vi "ActorPlugin-002-Inventory.vi"(0 "FTW Actor Instance Configuration":string="{\n  \"Identity\": \"ActorName\",\n  \"InboxAddress\": \"tcp://127.0.0.1:*\",\n  \"PublisherAddress\": \"tcp://127.0.0.1:*\",\n  \"DebugEnableInboxLogging\": false,\n  \"DebugEnableJobLogging\": false,\n  \"DebugShowPanel\": false\n}", 11 "Error":errorcluster) -> (15 "Error":errorcluster)   [LabVIEW 2013, in "ERP-Inventory.lvclass"]
uses:
  Actors/ERP-Inventory Plugin/ERP-Inventory.lvclass
  Inventory System/controls/Create Label Button.ctl
  Actors/ERP-Inventory Plugin/Inventory-Controls/Iventory-FinishedGoods.ctl
  Actors/ERP-Inventory Plugin/Inventory-Controls/Iventory-RawGoods.ctl
  Actors/ERP-Inventory Plugin/Inventory-Controls/Iventory-AdminOnly.ctl
  Actors/ERP-Inventory Plugin/ERP-Inventory.lvclass/ERP-Inventory.ctl
  <vilib>/Utility/error.llb/DialogType.ctl
  <vilib>/Utility/miscctls.llb/LVRowAndColumnUnsignedTypeDef.ctl
  ftw-dataflow/Actor/src/Instance/FTW-ActorInstance.lvclass
  ftw-dataflow/Actor/src/Message/Request/FTW-Message-IncomingRequest.lvclass
  ERP-ConfigPageNewFeather/PCert-ConfigPageNF.lvclass
panel:
  in  "Create Bag Label":T1
  in  "Admin":T2
  in  "Raw Goods":T3
  in  "Finished Goods":T4
  in  "Tab Control - Finished Goods":T5(tab)
  in  "Quanity to Add/Subtract":i32
  in  "Part Number to Search For":string
  in  "Refresh Finished Good List":bool
  in  "Clear Search":bool
  in  "Search Button":bool
  in  "Inventory Listbox":i32(listbox)
  in  "Add Finshed Goods":bool
  in  "Part Numbers":u16(ring) items=["", "------------Wafers---------------", "PC-1012MX", "PC-1015M", "PP-2015-7003SCM", "PP-2015-9903SC/I-M", "PP-2015-15003SCM", "PP-2023-7003SCM", "PP-2023-15003SCM", "PP-2023-30003SCM", "PL-5015-05AH", "PL-5015-1AH", "PL-5023-1AHG", "PF-4015-30003SCM", "PF-4022-30003SCM", "PF-4023-30003SCM", "PF-4043-30003SCM", "PF-4043-30015SCM", "-------Miscelaneous Parts-------", "TPR-CRP", "TPR-VRP", "TPR-LPF05", "TPR-LPF10", "TPR-VLPF-3SH", "PL-5001-1AH", "PP-2001-7003SCM", "PP-2001-9903SC/I-M", "PS-3001-1AHM", "PF-4001-30003SCM", "PP-2010-7003SCM", "PL-5010-1AH", "PS-3010-3AHM", "PF-4010-30015SCM", "PP-2049-30003SCM", "PP-2049-7003SCM", "PL-5049-1AH", "PP-2049-7003SCM", "PL-5044-1AH", "PL-5121-1AH", "PP-2055-7003SCM", "PL-5055-1AH", "PP-2129-7003SCM", "PL-5338-1AH", "PF-4014-30003SCM", "PF-4014-30010SCM", "PF-4008-30015SCM", "PF-4064-30015SCM", "PF-4111-30003SCM", "PF-4054-30003SCM", "NS-PP-2150-15003SCM", "CCW-7015-001-257-FL", "CCW-7015-01-150-FL", "CCW-7043-001-257-FL", "CCW-7043-01-150-FL", "Vacuum Chuck", "HHCR-12-1"]
  in  "Subtract Finished Goods":bool
  in  "Part Number to Search For Raw Goods":string caption="Part Number to Search For"
  in  "Subtract_Raw Goods":bool
  in  "Quanity to Add/Subtract_Raw Goods":i32 caption="Quanity to Add/Subtract"
  in  "Part Numbers_Raw Goods":u16(ring) caption="Part Numbers" items=["", "X042-MJC", "X042-IMFS", "X043-ITS", "X043J-ITS", "X022-ITS", "X023-ITS", "X016-MJC", "X094-ITS", "X094-TI", "X015-IMFT", "X015-MJC", "X015-ITS"]
  in  "Add Button_Raw Goods":bool
  in  "Raw Goods Listbox":i32(listbox)
  in  "Search Button_Raw Goods":bool
  in  "Clear Search_Raw Goods":bool
  in  "Refresh Raw Good List":bool
  in  "Tab Control - Delete Part Numbers":enum32{"Finsihed Goods", "Raw Goods"}(tab)
  in  "Delete Finished Good Part Number":bool
  in  "Finish Good Part# to Delete":u16(ring) caption="Part Numbers" items=["", "------------Wafers---------------", "PC-1012MX", "PC-1015M", "PP-2015-7003SCM", "PP-2015-9903SC/I-M", "PP-2015-15003SCM", "PP-2023-7003SCM", "PP-2023-15003SCM", "PP-2023-30003SCM", "PL-5015-05AH", "PL-5015-1AH", "PL-5023-1AHG", "PF-4015-30003SCM", "PF-4022-30003SCM", "PF-4023-30003SCM", "PF-4043-30003SCM", "PF-4043-30015SCM", "-------Miscelaneous Parts-------", "TPR-CRP", "TPR-VRP", "TPR-LPF05", "TPR-LPF10", "TPR-VLPF-3SH", "PL-5001-1AH", "PP-2001-7003SCM", "PP-2001-9903SC/I-M", "PS-3001-1AHM", "PF-4001-30003SCM", "PP-2010-7003SCM", "PL-5010-1AH", "PS-3010-3AHM", "PF-4010-30015SCM", "PP-2049-30003SCM", "PP-2049-7003SCM", "PL-5049-1AH", "PP-2049-7003SCM", "PL-5044-1AH", "PL-5121-1AH", "PP-2055-7003SCM", "PL-5055-1AH", "PP-2129-7003SCM", "PL-5338-1AH", "PF-4014-30003SCM", "PF-4014-30010SCM", "PF-4008-30015SCM", "PF-4064-30015SCM", "PF-4111-30003SCM", "PF-4054-30003SCM", "NS-PP-2150-15003SCM", "CCW-7015-001-257-FL", "CCW-7015-01-150-FL", "CCW-7043-001-257-FL", "CCW-7043-01-150-FL", "Vacuum Chuck", "HHCR-12-1"]
  in  "Raw Goods Part # to Delete":u16(ring) caption="Part Numbers" items=["", "X042-MJC", "X042-IMFS", "X043-ITS", "X043J-ITS", "X022-ITS", "X023-ITS", "X016-MJC", "X094-ITS", "X094-TI", "X015-IMFT", "X015-MJC", "X015-ITS"]
  in  "Delete Raw Good Part Number":bool
  in  "Maximum Number Allowed\nIn Inventory":i32
  in  "Minimum Number Allowed \nIn Inventory":i32
  in  "New Raw Good Part Number":bool
  in  "New Wafer Assembled Part?":bool
  in  "New Inventory Assembled Part Number to Add":string
  in  "Quanity to Add To Inventory New Part":i32
  out "String":string
  # "Inventory Controls"
  # "Inputs"
  # "Outputs"
  # "I am ready to run"
  # "Welcome to the ITS Inventory System\nPlease use the Inventory Controls below to \naccess the system."
  # "Finished Goods"
  # "Search Finished Goods DB"
  # "Add Part Number to Finished Goods"
  # "1."
  # "2."
  # "Raw Goods"
  # "Search Raw Goods DB"
  # "Add Part Number to Raw Goods"
  # "1."
  # "2."
  # "Admin Tools"
  # "Admin Add Parts to Database"
  # "Admin Delete Parts# From Database"
  # "Choose the Part Number that you would like to delete from the drop down menu. Then press delete."
  # "Choose the Part Number that you would like to delete from the drop down menu. Then press delete."
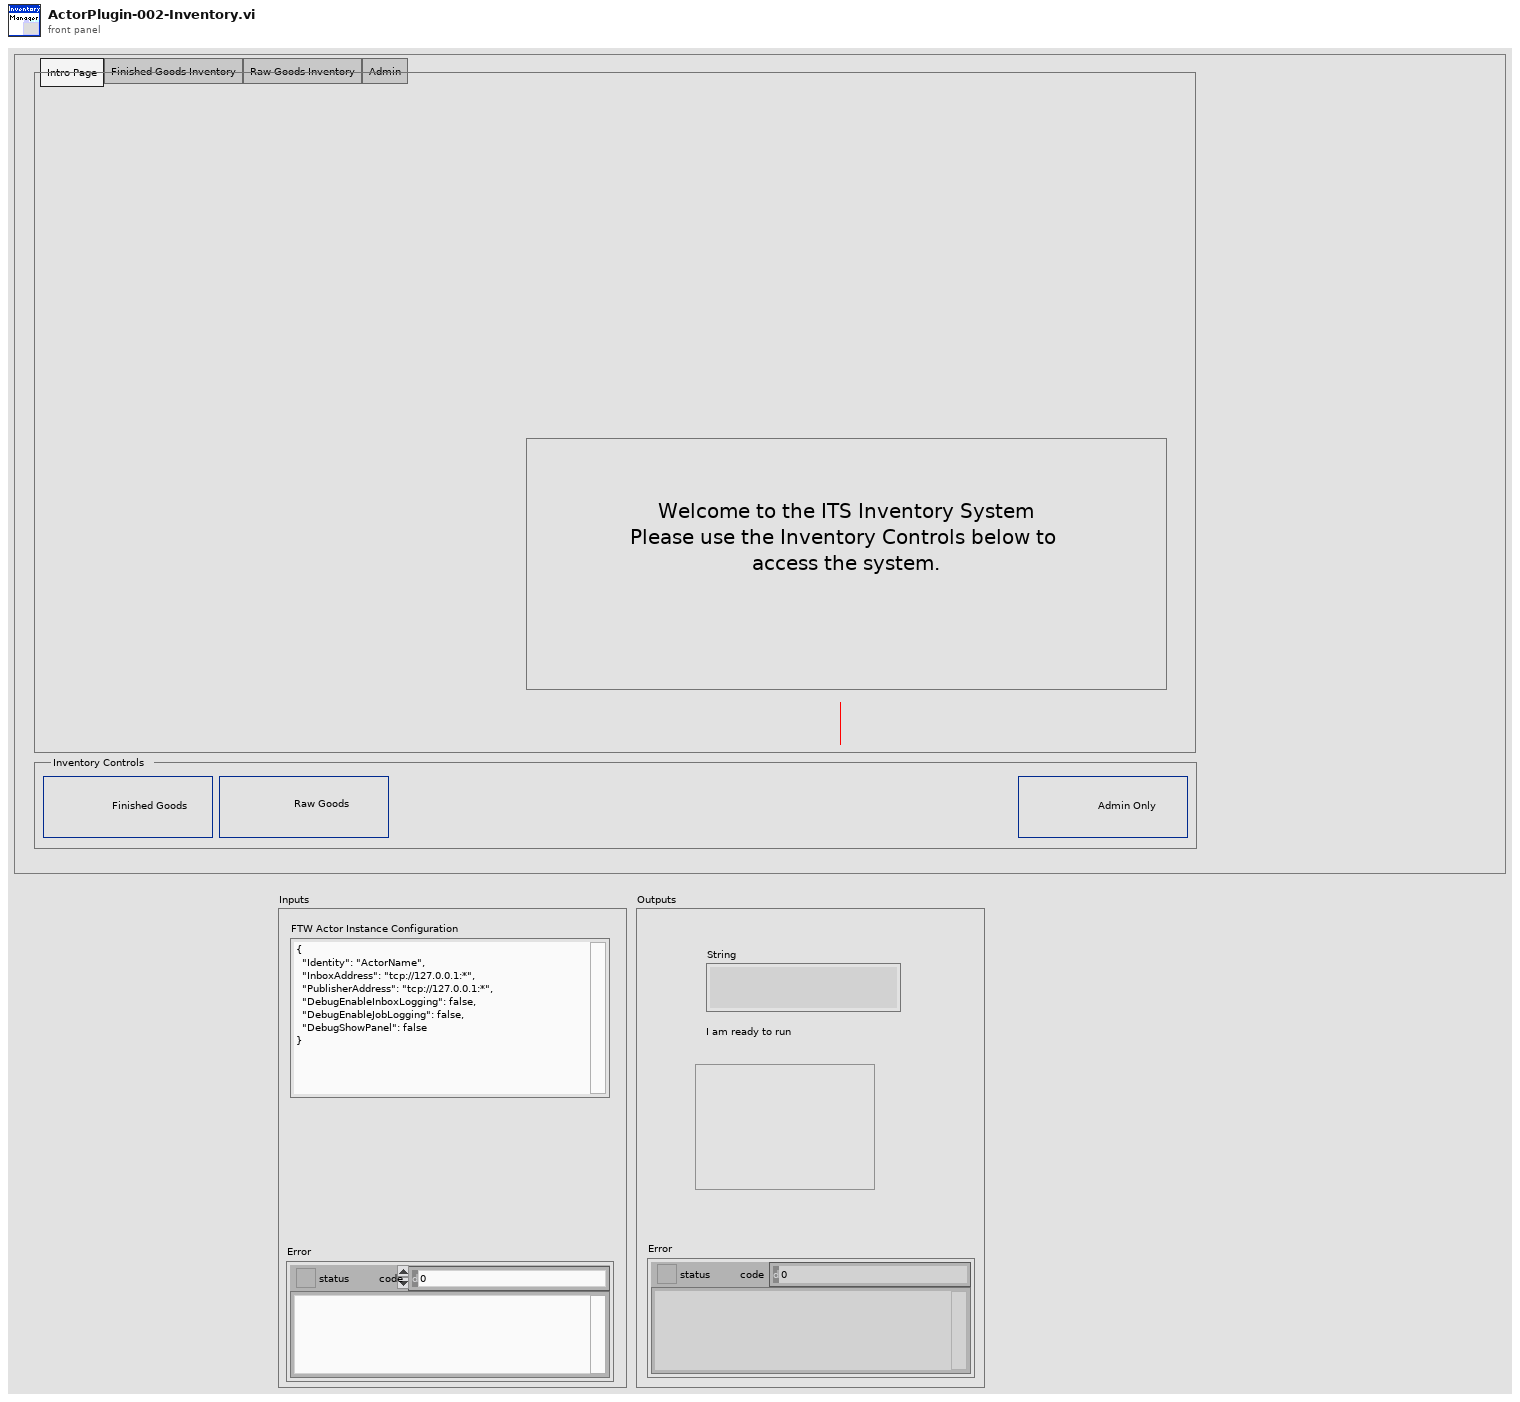
[diagram p1: front panel]
types:
  T1 = typedef "Create Label Button.ctl" = bool
  T2 = typedef "Iventory-AdminOnly.ctl" = bool
  T3 = typedef "Iventory-RawGoods.ctl" = bool
  T4 = typedef "Iventory-FinishedGoods.ctl" = bool
  T5 = enum32{"Intro Page", "Finished Goods Inventory", "Raw Goods Inventory", "Admin"}
  T6 = enum32{"Intro Page", "Finished Goods Inventory", "Raw Goods Inventory", "Inventory Waiting to be Stocked", "Fulfill Inventory Work Order", "Admin"}
  T7 = typedef "LVRowAndColumnUnsignedTypeDef.ctl" = cluster{"Row":u32, "Column":u32}
  T8 = cluster{"New Inventory Assembled Part Number to Add":string, "On the Shelf":string, "Minimum":string, "Maximum":string}
  T9 = typedef "DialogType.ctl" = u16
  T10 = cluster{"Incoming Requests":refnum<event-registration>, "Additional Registration Types":refnum<event-registration>}
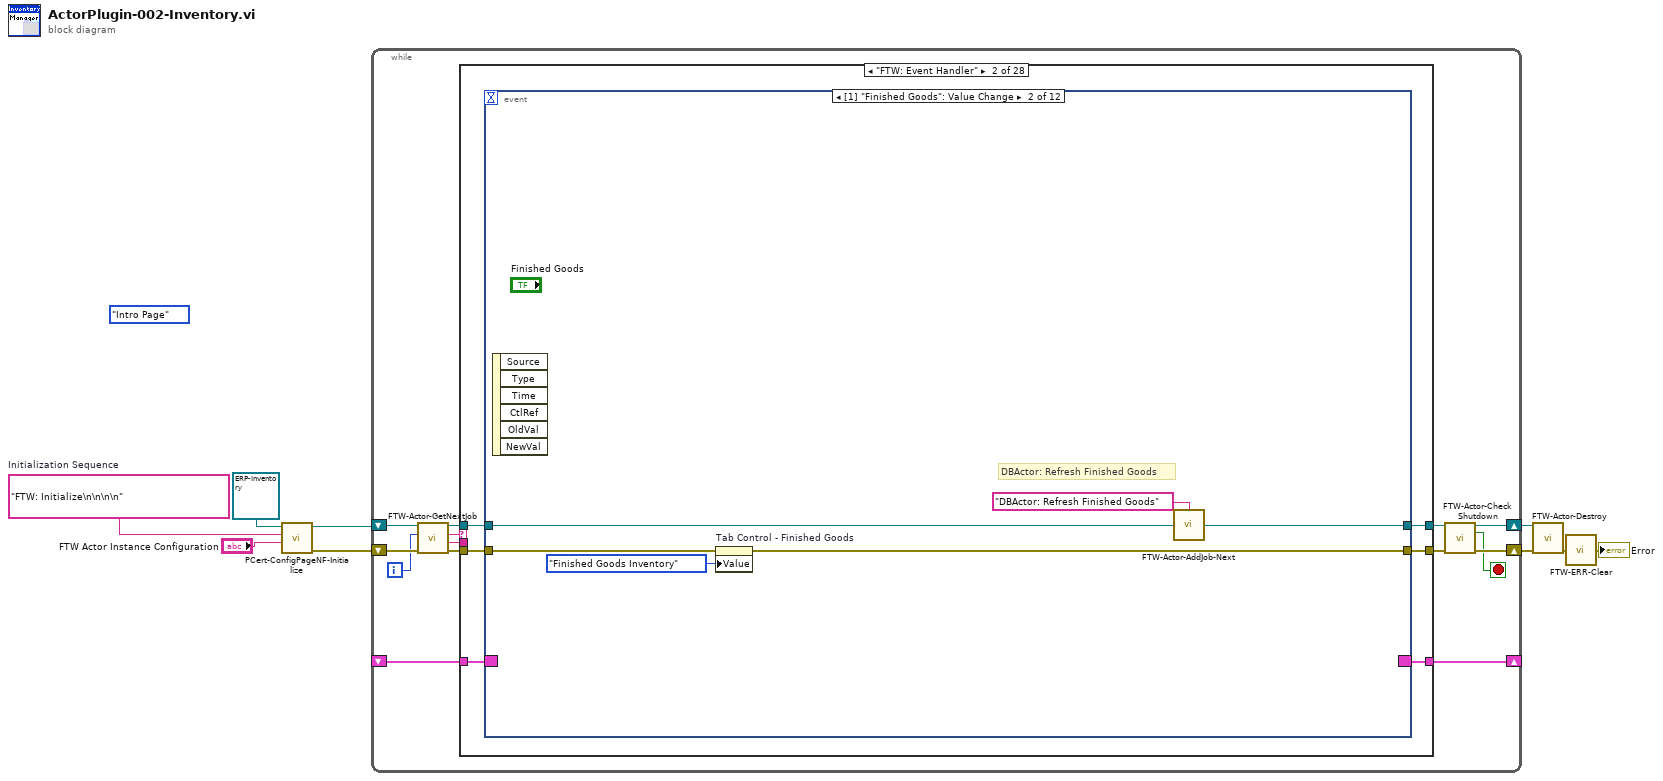
[diagram p0: block diagram]
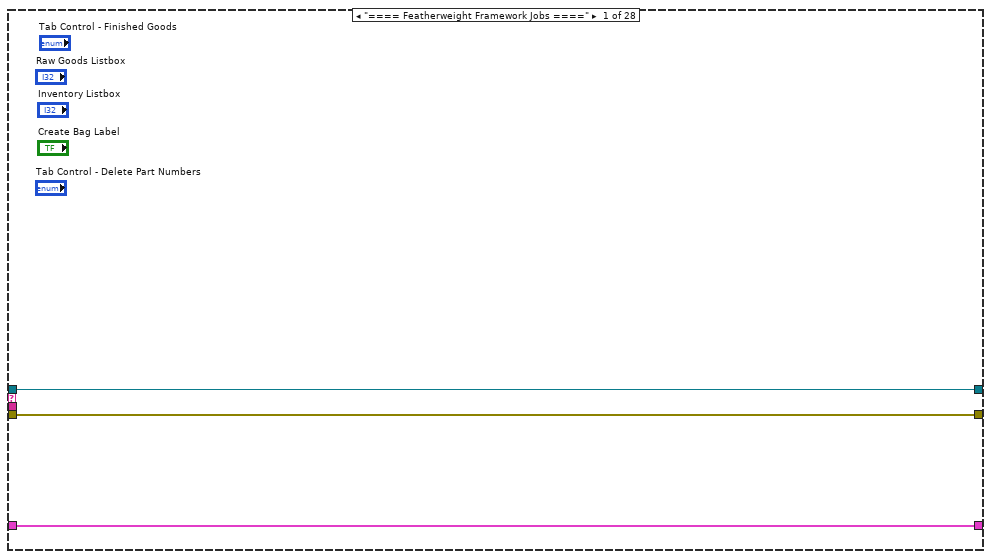
[diagram p2: hidden frame]
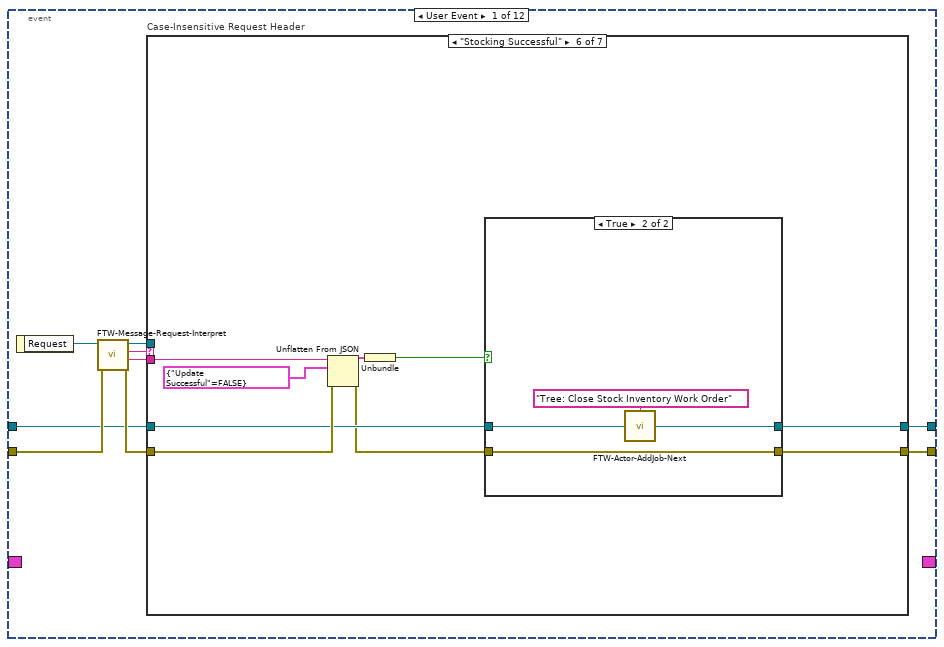
[diagram p3: hidden frame]
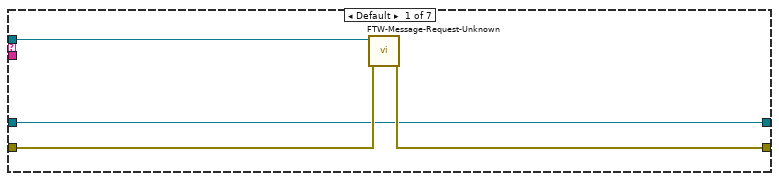
[diagram p4: hidden frame]
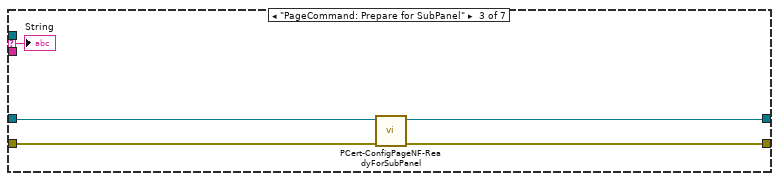
[diagram p6: hidden frame]
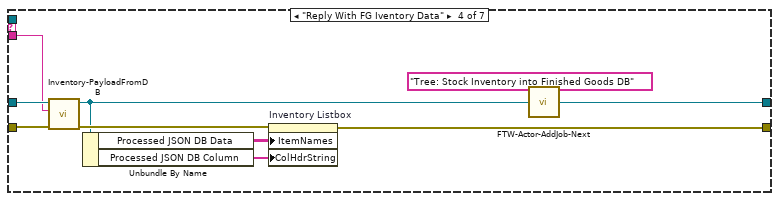
[diagram p7: hidden frame]
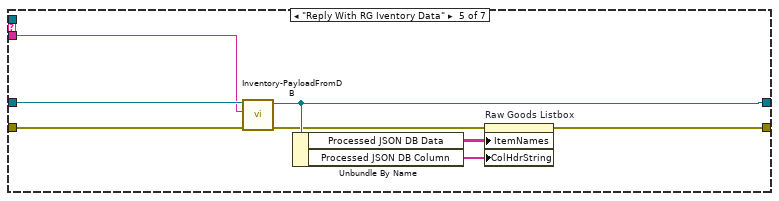
[diagram p8: hidden frame]
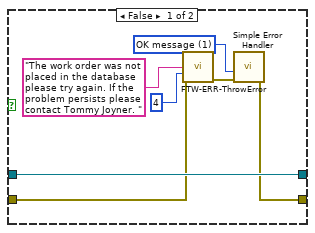
[diagram p9: hidden frame]
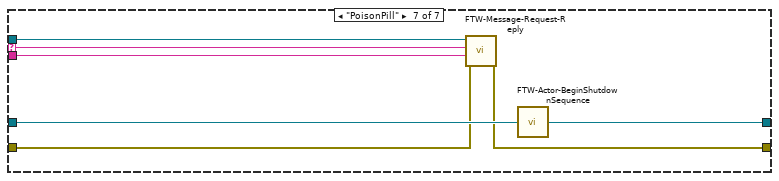
[diagram p10: hidden frame]
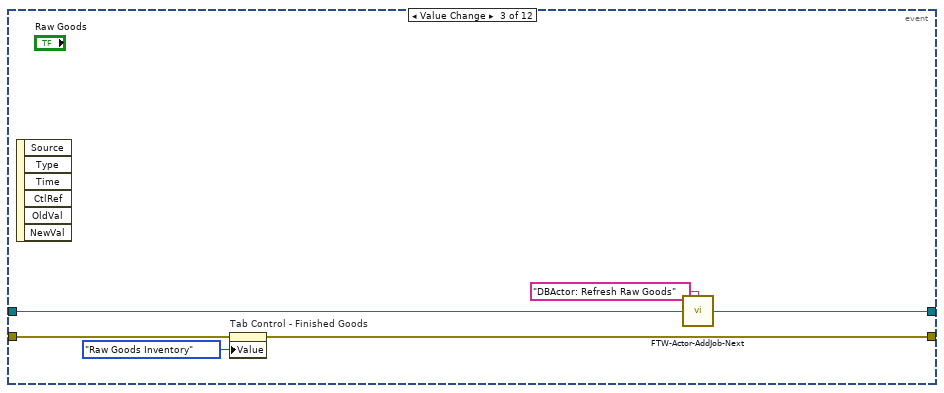
[diagram p11: hidden frame]
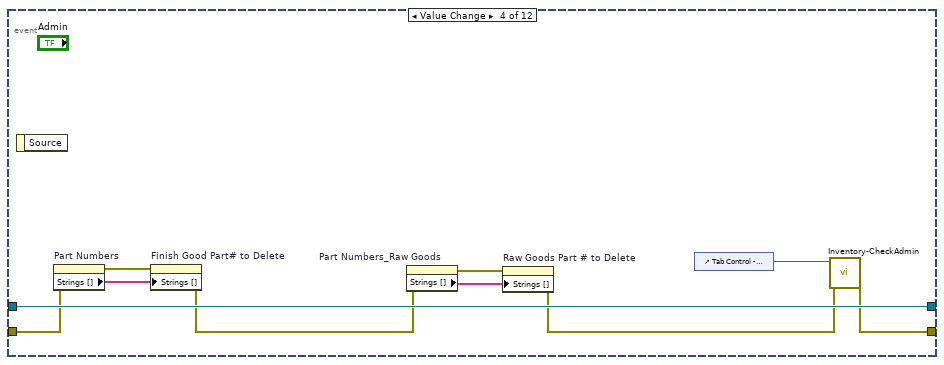
[diagram p12: hidden frame]
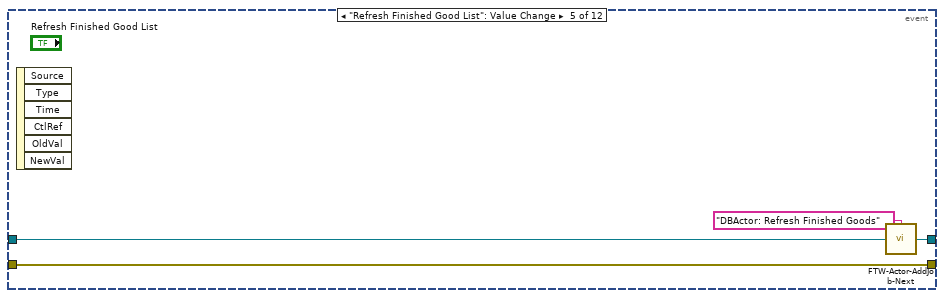
[diagram p13: hidden frame]
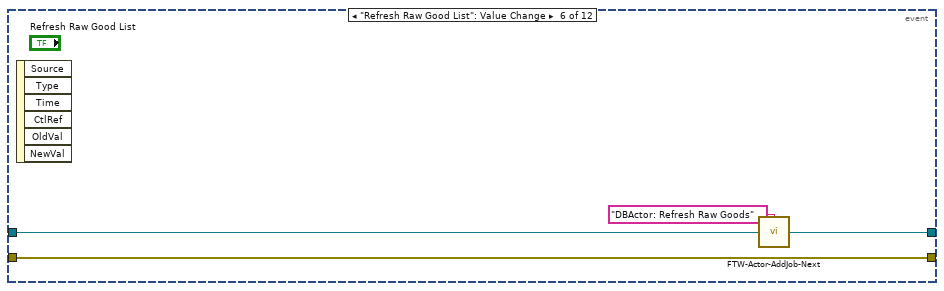
[diagram p14: hidden frame]
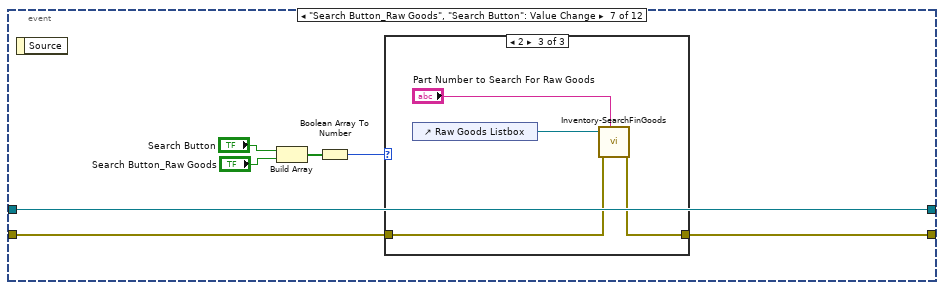
[diagram p15: hidden frame]
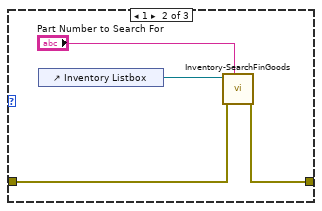
[diagram p17: hidden frame]
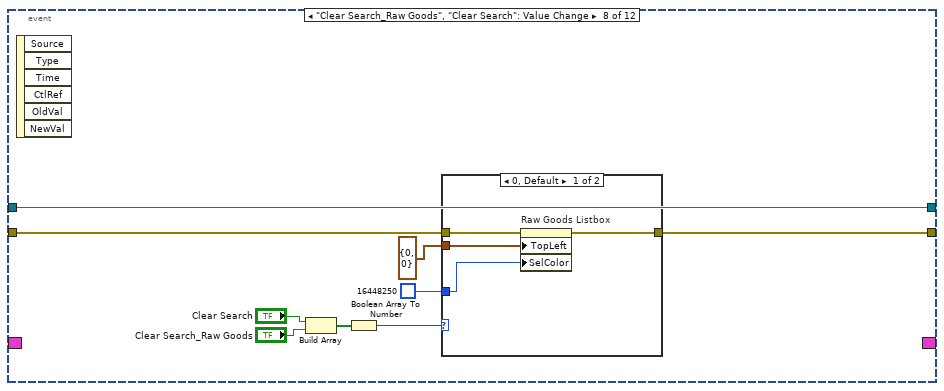
[diagram p18: hidden frame]
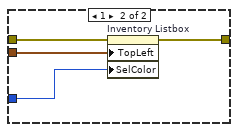
[diagram p19: hidden frame]
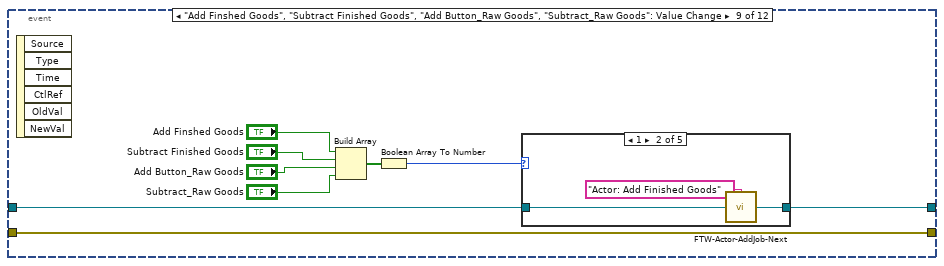
[diagram p20: hidden frame]
diagram:
  (unwired) T6."Intro Page" ("Tab Control - Finished Goods")
  w7 = "FTW: Initialize\n\n\n\n"  # Initialization Sequence
  n1 = call-dynamic "PCert-ConfigPageNF-Initialize.vi"("FTW Actor Instance Configuration"="FTW Actor Instance Configuration", "Initialization Job Sequence"=w7, "ERP-ConfigPageNF.lvclass"=refnum<class "ERP-Inventory.lvclass"> refnum ("ERP-Inventory.lvclass")) -> ("error out"=w5:errorcluster, "ERP-ConfigPageNF out"=w6:refnum<class "ERP-Inventory.lvclass">)  [unwired: 7 in]
  n2 = while {
    shift-right: [w13] -> w8
    shift-left: w5 -> [w20]
    shift-right: [w10] -> _
    shift-left: _ -> [w23]
    shift-right: [w15] -> w9
    shift-left: w6 -> [w22]
    i -> [w11]
    stop <- w12 stop-if-true
    n3 = call "FTW-Actor-GetNextJob.vi"("error in"=w20, "Jobs Performed"=w11, "FTW Actor Instance"=w22) -> ("error out"=w19:errorcluster, "Job Data"=w17:string, "Job Name"=w18:string, "FTW Actor Instance out"=w21:refnum<class "ERP-Inventory.lvclass">)  [unwired: 5 in]
    n4 = case shown="\"FTW: Event Handler\"" w18 {
      selector: w18 -> [_ _ _ _ w245 _ _ _ _ _ _ _ _ _ _ _ _ _ _ _ _ _ _ _ _ _ _ _]
      tunnel: [w25 w32 w238 w240 w248 w256 w262 w267 w271 w277 w292 w305 w320 w353 w386 w437 w486 w536 w566 w608 w632 w645 w648 w651 w654 w657 w660 w663] -> w14
      tunnel: w19 -> [w25 w31 w233 w242 w249 w252 w262 w267 w271 w283 w299 w314 w330 w342 w388 w439 w489 w558 w567 w604 w624 w645 w648 w651 w654 w657 w660 w663]
      tunnel: w23 -> [w26 w27 _ w244 w250 w258 w263 w268 w270 w287 w303 w319 w335 w361 w411 w461 w511 w565 w595 w619 w643 w646 w649 w652 w655 w658 w661 w664]
      tunnel: [w26 w30 w235 w244 w250 w258 w263 w268 w270 w287 w303 w319 w335 w361 w411 w461 w511 w565 w595 w619 w643 w646 w649 w652 w655 w658 w661 w664] -> w10
      tunnel: w17 -> [_ _ _ _ _ _ _ _ _ _ _ _ _ _ _ _ _ _ _ _ _ _ _ _ _ _ _ _]
      tunnel: [w24 w29 w239 w241 w246 w253 w260 w265 w269 w272 w288 w304 w321 w354 w387 w436 w487 w564 w568 w609 w633 w644 w647 w650 w653 w656 w659 w662] -> w16
      tunnel: w21 -> [w24 w28 w234 w243 w247 w254 w261 w266 w269 w279 w293 w309 w326 w360 w389 w438 w488 w559 w569 w610 w634 w644 w647 w650 w653 w656 w659 w662]
      frame "==== Featherweight Framework Jobs ====" {
      }
      frame "FTW: Event Handler" {
        n5 = event shown="[1] \"Finished Goods\": Value Change" {
          selector: w27 -> [_ _ _ _ _ _ _ _ _ _ _ _]
          dyn-events: [_ _ _ _ _ _ _ _ _ _ _ _] -> w30
          timeout: _ -> [_ _ _ _ _ _ _ _ _ _ _ _]
          tunnel: [w38 w102 w108 w118 w123 w127 w132 w150 w169 w183 w217 w227] -> w32
          tunnel: w31 -> [w39 w103 w109 w114 w123 w127 w133 w151 w169 w189 w217 w227]
          tunnel: [w37 w101 w106 w119 w121 w125 w134 w152 w161 w194 w213 w225] -> w29
          tunnel: w28 -> [w36 w99 w105 w119 w120 w124 w134 w152 w162 w200 w214 w226]
          event User Event {
            n6 = event-data() -> ("Request"=w40:refnum<class "FTW-Message-IncomingRequest.lvclass">)  [unwired: 1 in]
            n7 = call "FTW-Message-Request-Interpret.vi"("error in"=w39, "FTW Incoming Request"=w40) -> ("error out"=w41:errorcluster, "Request Body"=w34:string, "Request Header"=w35:string, "FTW Incoming Request out"=w33:refnum<class "FTW-Message-IncomingRequest.lvclass">)  [unwired: 6 in]
            n8 = case "Case-Insensitive Request Header" shown="\"Stocking Successful\"" w35 {
              selector: w35 -> [_ _ w48 _ _ _ w93]
              tunnel: [w44 w46 w50 w62 w66 w71 w91] -> w38
              tunnel: w41 -> [w45 w46 w52 w60 w69 w78 w92]
              tunnel: [w42 w47 w49 w54 w68 w73 w97] -> w37
              tunnel: w36 -> [w42 w47 w51 w61 w70 w74 w96]
              tunnel: w34 -> [_ _ _ w53 w63 w79 w94]
              tunnel: w33 -> [w43 _ _ _ _ _ w95]
              frame Default {
                n9 = call "FTW-Message-Request-Unknown.vi"("error in"=w45, "FTW Incoming Request"=w43) -> ("error out"=w44:errorcluster)  [unwired: 9 in]
              }
              frame "Cold Call Success" {
              }
              frame "PageCommand: Prepare for SubPanel" {
                n10 = call "PCert-ConfigPageNF-ReadyForSubPanel.vi"("error in (no error)"=w52, "ERP-ConfigPageNF in"=w51) -> ("error out"=w50:errorcluster, "ERP-ConfigPageNF out"=w49:refnum<class "ERP-Inventory.lvclass">)  [unwired: 8 in]
                "String" <- w48
              }
              frame "Reply With FG Iventory Data" {
                n11 = call "Inventory-PayloadFromDB.vi"("error in (no error)"=w60, "JSON string"=w53, "ERP-Inventory in"=w61) -> ("error out"=w59:errorcluster, "ERP-Inventory out"=w55:refnum<class "ERP-Inventory.lvclass">)  [unwired: 7 in]
                n12 = Unbundle By Name(w55) -> ("Processed JSON DB Data"=w58:string[][], "Processed JSON DB Column"=w57:string[])
                n13 = property on="Inventory Listbox" class="MCListbox (strict)"(error in=w59, "ItemNames"=w58, "ColHdrString"=w57) -> (error out=w62:errorcluster)  [unwired: 1 in, 1 out]
                n14 = call "FTW-Actor-AddJob-Next.vi"("Add Next in Job Queue"="Tree: Stock Inventory into Finished Goods DB", "FTW Actor Instance"=w55) -> ("FTW Actor Instance out"=w54:refnum<class "ERP-Inventory.lvclass">)  [unwired: 2 in]
              }
              frame "Reply With RG Iventory Data" {
                n15 = call "Inventory-PayloadFromDB.vi"("error in (no error)"=w69, "JSON string"=w63, "ERP-Inventory in"=w70) -> ("error out"=w67:errorcluster, "ERP-Inventory out"=w68:refnum<class "ERP-Inventory.lvclass">)  [unwired: 7 in]
                n16 = Unbundle By Name(w68) -> ("Processed JSON DB Data"=w65:string[][], "Processed JSON DB Column"=w64:string[])
                n17 = property on="Raw Goods Listbox" class="MCListbox (strict)"(error in=w67, "ItemNames"=w65, "ColHdrString"=w64) -> (error out=w66:errorcluster)  [unwired: 1 in, 1 out]
              }
              frame "Stocking Successful" {
                n18 = Unflatten From JSON(JSON string=w79, type and defaults=cluster{"Update Successful":bool} {"Update Successful"=FALSE}, error in (no error)=w78) -> (value=w76:cluster{"Update Successful":bool}, error out=w72:errorcluster)  [unwired: 4 in]
                n19 = Unbundle(w76) -> ("Update Successful"=w75:bool)
                n20 = case shown="True" w75 {
                  tunnel: w74 -> [w86 w89]
                  tunnel: [w86 w88] -> w73
                  tunnel: w72 -> [w82 w87]
                  tunnel: [w81 w87] -> w71
                  frame False {
                    w83 = T9 1 items=["no dialog", "OK message", "continue or stop message", "OK message + warnings", "continue/stop + warnings"] ("type of dialog (OK msg:1)")
                    n21 = call "FTW-ERR-ThrowError.vi"("Error Message"="The work order was not placed in the database please try again. If the problem persists please contact Tommy Joyner. ", "Error Code"=4, "error in"=w82) -> ("error out"=w84:errorcluster)  [unwired: 12 in]
                    n22 = call <vilib>:"Simple Error Handler.vi"("type of dialog (OK msg:1)"=w83, "error in (no error)"=w84) -> ("error out"=w81:errorcluster)  [unwired: 3 in, 4 out]
                  }
                  frame True {
                    n23 = call "FTW-Actor-AddJob-Next.vi"("Add Next in Job Queue"="Tree: Close Stock Inventory Work Order", "FTW Actor Instance"=w89) -> ("FTW Actor Instance out"=w88:refnum<class "ERP-Inventory.lvclass">)  [unwired: 2 in]
                  }
                }
              }
              frame "PoisonPill" {
                n24 = call "FTW-Message-Request-Reply.vi"("error in"=w92, "Response Body"=w94, "Response Header"=w93, "FTW Incoming Request"=w95) -> ("error out"=w91:errorcluster)  [unwired: 6 in, 1 out]
                n25 = call "FTW-Actor-BeginShutdownSequence.vi"("FTW Actor Instance"=w96) -> ("FTW Actor Instance out"=w97:refnum<class "ERP-Inventory.lvclass">)  [unwired: 3 in]
              }
            }
          }
          event Value Change {
            # "DBActor: Refresh Finished Goods"
            n26 = event-data() -> ()  [unwired: 1 in, 6 out]
            n27 = property on="Tab Control - Finished Goods" class="TabCtl (strict)"(error in=w103, "Value"=T5."Finished Goods Inventory" ("Tab Control - Finished Goods")) -> (error out=w102:errorcluster)  [unwired: 1 in, 1 out]
            n28 = call "FTW-Actor-AddJob-Next.vi"("Add Next in Job Queue"="DBActor: Refresh Finished Goods", "FTW Actor Instance"=w99) -> ("FTW Actor Instance out"=w101:refnum<class "ERP-Inventory.lvclass">)  [unwired: 2 in]
          }
          event Value Change {
            n29 = event-data() -> ()  [unwired: 1 in, 6 out]
            n30 = property on="Tab Control - Finished Goods" class="TabCtl (strict)"(error in=w109, "Value"=T5."Raw Goods Inventory" ("Tab Control - Finished Goods")) -> (error out=w108:errorcluster)  [unwired: 1 in, 1 out]
            n31 = call "FTW-Actor-AddJob-Next.vi"("Add Next in Job Queue"="DBActor: Refresh Raw Goods", "FTW Actor Instance"=w105) -> ("FTW Actor Instance out"=w106:refnum<class "ERP-Inventory.lvclass">)  [unwired: 2 in]
          }
          event Value Change {
            n32 = event-data() -> ()  [unwired: 1 in, 1 out]
            n33 = property on="Part Numbers" class="Ring (strict)"(error in=w114) -> (error out=w115:errorcluster, "Strings []"=w116:string[])  [unwired: 1 in, 1 out]
            n34 = property on="Finish Good Part# to Delete" class="Ring (strict)"(error in=w115, "Strings []"=w116) -> (error out=w112:errorcluster)  [unwired: 1 in, 1 out]
            n35 = property on="Part Numbers_Raw Goods" class="Ring (strict)"(error in=w112) -> (error out=w113:errorcluster, "Strings []"=w117:string[])  [unwired: 1 in, 1 out]
            n36 = property on="Raw Goods Part # to Delete" class="Ring (strict)"(error in=w113, "Strings []"=w117) -> (error out=w111:errorcluster)  [unwired: 1 in, 1 out]
            n37 = control-ref of="Tab Control - Finished Goods"() -> (w110:refnum<vi>)
            n38 = call "Inventory-CheckAdmin.vi"("error in (no error)"=w111, "Tab Control - Finished Goods"=w110) -> ("error out"=w118:errorcluster)  [unwired: 9 in]
          }
          event "Refresh Finished Good List": Value Change {
            n39 = event-data() -> ()  [unwired: 1 in, 6 out]
            n40 = call "FTW-Actor-AddJob-Next.vi"("Add Next in Job Queue"="DBActor: Refresh Finished Goods", "FTW Actor Instance"=w120) -> ("FTW Actor Instance out"=w121:refnum<class "ERP-Inventory.lvclass">)  [unwired: 2 in]
          }
          event "Refresh Raw Good List": Value Change {
            n41 = event-data() -> ()  [unwired: 1 in, 6 out]
            n42 = call "FTW-Actor-AddJob-Next.vi"("Add Next in Job Queue"="DBActor: Refresh Raw Goods", "FTW Actor Instance"=w124) -> ("FTW Actor Instance out"=w125:refnum<class "ERP-Inventory.lvclass">)  [unwired: 2 in]
          }
          event "Search Button_Raw Goods", "Search Button": Value Change {
            n43 = event-data() -> ()  [unwired: 1 in, 1 out]
            n44 = Build Array("Search Button", "Search Button_Raw Goods") -> (w129:bool[])
            n45 = Boolean Array To Number(Boolean array=w129) -> (number=w128:u32)
            n46 = case shown="2" w128 {
              tunnel: w133 -> [w135 w139 w143]
              tunnel: [w135 w138 w142] -> w132
              frame 0, Default {
              }
              frame 1 {
                n47 = control-ref of="Inventory Listbox"() -> (w137:refnum<vi>)
                n48 = call "Inventory-SearchFinGoods.vi"("Part Number to Search For"="Part Number to Search For", "error in (no error)"=w139, "Inventory Listbox"=w137) -> ("error out"=w138:errorcluster)  [unwired: 8 in]
              }
              frame 2 {
                n49 = control-ref of="Raw Goods Listbox"() -> (w140:refnum<vi>)
                n50 = call "Inventory-SearchFinGoods.vi"("Part Number to Search For"="Part Number to Search For Raw Goods", "error in (no error)"=w143, "Inventory Listbox"=w140) -> ("error out"=w142:errorcluster)  [unwired: 8 in]
              }
            }
          }
          event "Clear Search_Raw Goods", "Clear Search": Value Change {
            n51 = event-data() -> ()  [unwired: 1 in, 6 out]
            n52 = Build Array("Clear Search", "Clear Search_Raw Goods") -> (w147:bool[])
            n53 = Boolean Array To Number(Boolean array=w147) -> (number=w144:u32)
            n54 = case shown="0, Default" w144 {
              tunnel: w151 -> [w156 w160]
              tunnel: [w155 w159] -> w150
              tunnel: T7 {"Row"=0, "Column"=0} ("Top Left Visible Cell") -> [w154 w158]
              tunnel: u32 16448250 -> [w153 w157]
              frame 0, Default {
                n55 = property on="Raw Goods Listbox" class="MCListbox (strict)"(error in=w156, "TopLeft"=w154, "SelColor"=w153) -> (error out=w155:errorcluster)  [unwired: 1 in, 1 out]
              }
              frame 1 {
                n56 = property on="Inventory Listbox" class="MCListbox (strict)"(error in=w160, "TopLeft"=w158, "SelColor"=w157) -> (error out=w159:errorcluster)  [unwired: 1 in, 1 out]
              }
            }
          }
          event "Add Finshed Goods", "Subtract Finished Goods", "Add Button_Raw Goods", "Subtract_Raw Goods": Value Change {
            n57 = event-data() -> ()  [unwired: 1 in, 6 out]
            n58 = Build Array("Add Finshed Goods", "Subtract Finished Goods", "Add Button_Raw Goods", "Subtract_Raw Goods") -> (w164:bool[])
            n59 = Boolean Array To Number(Boolean array=w164) -> (number=w163:u32)
            n60 = case shown="1" w163 {
              tunnel: w162 -> [w170 w173 w176 w179 w182]
              tunnel: [w170 w171 w174 w177 w180] -> w161
              frame 0, Default {
              }
              frame 1 {
                n61 = call "FTW-Actor-AddJob-Next.vi"("Add Next in Job Queue"="Actor: Add Finished Goods", "FTW Actor Instance"=w173) -> ("FTW Actor Instance out"=w171:refnum<class "ERP-Inventory.lvclass">)  [unwired: 2 in]
              }
              frame 2 {
                n62 = call "FTW-Actor-AddJob-Next.vi"("Add Next in Job Queue"="Actor: Subtract Finished Goods", "FTW Actor Instance"=w176) -> ("FTW Actor Instance out"=w174:refnum<class "ERP-Inventory.lvclass">)  [unwired: 2 in]
              }
              frame 4 {
                n63 = call "FTW-Actor-AddJob-Next.vi"("Add Next in Job Queue"="Actor: Add Raw Goods", "FTW Actor Instance"=w179) -> ("FTW Actor Instance out"=w177:refnum<class "ERP-Inventory.lvclass">)  [unwired: 2 in]
              }
              frame 8 {
                n64 = call "FTW-Actor-AddJob-Next.vi"("Add Next in Job Queue"="Actor: Subtract Raw Goods", "FTW Actor Instance"=w182) -> ("FTW Actor Instance out"=w180:refnum<class "ERP-Inventory.lvclass">)  [unwired: 2 in]
              }
            }
          }
          event "New Wafer Assembled Part?", "New Inventory Assembled Part Number to Add": Value Change {
            n65 = event-data() -> ()  [unwired: 1 in, 6 out]
            n66 = Build Array("New Wafer Assembled Part?", "New Raw Good Part Number") -> (w197:bool[])
            n67 = Boolean Array To Number(Boolean array=w197) -> (number=w196:u32)
            n68 = case shown="1" w196 {
              tunnel: w200 -> [w202 w205 w209]
              tunnel: [w202 w204 w208] -> w195
              tunnel: w189 -> [w201 w203 w207]
              tunnel: [w201 w203 w207] -> w184
              frame 0, Default {
              }
              frame 1 {
                n69 = call "FTW-Actor-AddJob-Next.vi"("Add Next in Job Queue"="Actor: Add New Finished Goods Part#", "FTW Actor Instance"=w205) -> ("FTW Actor Instance out"=w204:refnum<class "ERP-Inventory.lvclass">)  [unwired: 2 in]
              }
              frame 2 {
                n70 = call "FTW-Actor-AddJob-Next.vi"("Add Next in Job Queue"="Actor: Add New Raw Goods Part#", "FTW Actor Instance"=w209) -> ("FTW Actor Instance out"=w208:refnum<class "ERP-Inventory.lvclass">)  [unwired: 2 in]
              }
            }
            n71 = Bundle By Name(cluster=w195, "New Inventory Assembled Part Number to Add"="New Inventory Assembled Part Number to Add", "Quanity to Add To Inventory New Part"="Quanity to Add To Inventory New Part", "Minimum Number Allowed \nIn Inventory"="Minimum Number Allowed \nIn Inventory", "Maximum Number Allowed\nIn Inventory"="Maximum Number Allowed\nIn Inventory") -> (w194:refnum<class "ERP-Inventory.lvclass">)
            n72 = invoke on="Minimum Number Allowed \nIn Inventory" class="DigNum (strict)" method="Reinit To Default"(error in=w184) -> (error out=w186:errorcluster)  [unwired: 2 in, 2 out]
            n73 = invoke on="Maximum Number Allowed\nIn Inventory" class="DigNum (strict)" method="Reinit To Default"(error in=w184) -> (error out=w185:errorcluster)  [unwired: 2 in, 2 out]
            n74 = invoke on="New Inventory Assembled Part Number to Add" class="Str" method="Reinit To Default"(error in=w184) -> (error out=w188:errorcluster)  [unwired: 2 in, 2 out]
            n75 = invoke on="Quanity to Add To Inventory New Part" class="DigNum (strict)" method="Reinit To Default"(error in=w184) -> (error out=w187:errorcluster)  [unwired: 2 in, 2 out]
            n76 = Merge Errors(w188, w187, w186, w185) -> (w183:errorcluster)
          }
          event "Delete Finished Good Part Number", "Delete Raw Good Part Number": Value Change {
            n77 = event-data() -> ()  [unwired: 1 in, 6 out]
            n78 = Build Array("Delete Finished Good Part Number", "Delete Raw Good Part Number") -> (w216:bool[])
            n79 = Boolean Array To Number(Boolean array=w216) -> (number=w215:u32)
            n80 = case shown="2" w215 {
              tunnel: w214 -> [w218 w220 w223]
              tunnel: [w218 w219 w222] -> w213
              frame 0, Default {
              }
              frame 1 {
                n81 = call "FTW-Actor-AddJob-Next.vi"("Add Next in Job Queue"="Actor: Delete Finished Goods Part#", "FTW Actor Instance"=w220) -> ("FTW Actor Instance out"=w219:refnum<class "ERP-Inventory.lvclass">)  [unwired: 2 in]
              }
              frame 2 {
                n82 = call "FTW-Actor-AddJob-Next.vi"("Add Next in Job Queue"="Actor: Delete Raw Goods Part#", "FTW Actor Instance"=w223) -> ("FTW Actor Instance out"=w222:refnum<class "ERP-Inventory.lvclass">)  [unwired: 2 in]
              }
            }
          }
          event Panel Close? {
            n83 = event-data() -> ()  [unwired: 1 in, 1 out]
            n84 = call "FTW-Actor-BeginShutdownSequence.vi"("FTW Actor Instance"=w226) -> ("FTW Actor Instance out"=w225:refnum<class "ERP-Inventory.lvclass">)  [unwired: 3 in]
            n85 = event-data("Discard?"=TRUE) -> ()  [unwired: 1 in, 1 out]
          }
        }
      }
      frame "FTW: Initialize" {
        w237 = refnum<event-registration> refnum  # Additional Registration Types
        n86 = property on="Tab Control - Finished Goods" class="TabCtl (strict)"(error in=w233, "Value"=T5."Intro Page" ("Tab Control - Finished Goods")) -> (error out=w232:errorcluster)  [unwired: 1 in, 1 out]
        n87 = call "PCert-ConfigPageNF-InRequests.vi"("error in (no error)"=w232, "ERP-ConfigPageNF in"=w234) -> ("error out"=w230:errorcluster, "Incoming Requests"=w236:refnum<event-registration>, "ERP-ConfigPageNF out"=w231:refnum<class "ERP-Inventory.lvclass">)  [unwired: 7 in]
        n88 = Bundle("Incoming Requests"=w236, "Additional Registration Types"=w237) -> (w235:T10)  [unwired: 1 in]
        n89 = call-dynamic "FTW-Actor-Initialized.vi"("FTW Actor Instance"=w231, "error in"=w230) -> ("FTW Actor Instance out"=w239:refnum<class "ERP-Inventory.lvclass">, "error out"=w238:errorcluster)  [unwired: 12 in]
      }
      frame "FTW: Error Handler" {
        n90 = call-dynamic "FTW-Actor-HandleError.vi"("FTW Actor Instance"=w243, "error in"=w242) -> ("FTW Actor Instance out"=w241:refnum<class "ERP-Inventory.lvclass">, "error out"=w240:errorcluster)  [unwired: 11 in, 1 out]
      }
      frame "FTW: Unknown Job", Default {
        n91 = call-dynamic "FTW-Actor-UnknownJob.vi"("FTW Actor Instance"=w247, "Unknown Job"=w245, "error in"=w249) -> ("FTW Actor Instance out"=w246:refnum<class "ERP-Inventory.lvclass">, "error out"=w248:errorcluster)  [unwired: 11 in]
      }
      frame "FTW: Shutdown" {
        n92 = call "PCert-ConfigPageNF-CloseActorConn.vi"("error in (no error)"=w252, "ERP-ConfigPageNF in"=w254) -> ("error out"=w251:errorcluster, "ERP-ConfigPageNF out"=w253:refnum<class "ERP-Inventory.lvclass">)  [unwired: 8 in]
        n93 = Unbundle(w258) -> ("Incoming Requests"=w257:refnum<event-registration>)  [unwired: 1 out]
        n94 = Unregister For Events(event registration refnum=w257) -> (error out=w255:errorcluster)  [unwired: 1 in]
        n95 = Merge Errors(w251, w255) -> (w256:errorcluster)
      }
      frame "FTW Sequence: Shutdown" {
        w259 = "FTW: Shutdown"  # Shutdown Sequence
        n96 = call "FTW-Actor-AddJob-Next.vi"("Add Next in Job Queue"=w259, "FTW Actor Instance"=w261) -> ("FTW Actor Instance out"=w260:refnum<class "ERP-Inventory.lvclass">)  [unwired: 2 in]
      }
      frame "==== Actor-Specific Job Sequences ====" {
        w264 = ""  # Job Sequence
        n97 = call "FTW-Actor-AddJob-Next.vi"("Add Next in Job Queue"=w264, "FTW Actor Instance"=w266) -> ("FTW Actor Instance out"=w265:refnum<class "ERP-Inventory.lvclass">)  [unwired: 2 in]
      }
      frame "==== Actor-Specific Jobs ====" {
      }
      frame "DBActor: Refresh Finished Goods" {
        w286 = ""
        n98 = call "JSON-ActorCommand.vi"("Payload"=w286, "error in"=w283, "Reply Command"="ReplyWithQuery" ("Value"), "SQL Statement"=w286, "Table"="Inventory") -> ("error out"=w280:errorcluster, "Output JSON Object"=w281:string)  [unwired: 5 in]
        n99 = call "PCert-ConfigPageNF-AskDB.vi"("Timeout"=500, "error in (no error)"=w280, "Request Body"=w281, "Request Header"="Query" ("Message Header"), "ERP-ConfigPageNF in"=w279) -> ("error out"=w278:errorcluster, "ERP-ConfigPageNF out"=w273:refnum<class "ERP-Inventory.lvclass">, "Raw Column Data From DB"=w274:string[], "Raw Data From DB"=w275:string[][])  [unwired: 2 in, 1 out]
        n100 = property on="Inventory Listbox" class="MCListbox (strict)"(error in=w278, "ItemNames"=w275, "ColHdrString"=w274) -> (error out=w277:errorcluster)  [unwired: 1 in, 1 out]
        n101 = Bundle By Name(cluster=w273, "Processed JSON DB Data"=w275, "Processed JSON DB Column"=w274) -> (w272:refnum<class "ERP-Inventory.lvclass">)
      }
      frame "DBActor: Refresh Raw Goods" {
        w302 = ""
        n102 = call "JSON-ActorCommand.vi"("Payload"=w302, "error in"=w299, "Reply Command"="ReplyWithQuery" ("Value"), "SQL Statement"=w302, "Table"="RawGoodInventory") -> ("error out"=w296:errorcluster, "Output JSON Object"=w294:string)  [unwired: 5 in]
        n103 = call "PCert-ConfigPageNF-AskDB.vi"("Timeout"=500, "error in (no error)"=w296, "Request Body"=w294, "Request Header"="Query" ("Message Header"), "ERP-ConfigPageNF in"=w293) -> ("error out"=w295:errorcluster, "ERP-ConfigPageNF out"=w289:refnum<class "ERP-Inventory.lvclass">, "Raw Column Data From DB"=w291:string[], "Raw Data From DB"=w290:string[][])  [unwired: 2 in, 1 out]
        n104 = property on="Raw Goods Listbox" class="MCListbox (strict)"(error in=w295, "ItemNames"=w290, "ColHdrString"=w291) -> (error out=w292:errorcluster)  [unwired: 1 in, 1 out]
        n105 = Bundle By Name(cluster=w289, "Processed JSON DB Data"=w290, "Processed JSON DB Column"=w291) -> (w288:refnum<class "ERP-Inventory.lvclass">)
      }
      frame "DBActor: Refresh Stock Inventory" {
        n106 = call "JSON-ActorCommand.vi"("Payload"="", "error in"=w314, "Reply Command"="ReplyWithQuery" ("Value"), "SQL Statement"="Where Status='Ready For Stocking'" ("Value"), "Table"="WorkOrders") -> ("error out"=w311:errorcluster, "Output JSON Object"=w310:string)  [unwired: 5 in]
        n107 = call "PCert-ConfigPageNF-AskDB.vi"("Timeout"=500, "error in (no error)"=w311, "Request Body"=w310, "Request Header"="Query" ("Message Header"), "ERP-ConfigPageNF in"=w309) -> ("error out"=w307:errorcluster, "ERP-ConfigPageNF out"=w308:refnum<class "ERP-Inventory.lvclass">, "Raw Data From DB"=w306:string[][])  [unwired: 2 in, 2 out]
        n108 = call "Inventory-StockTree.vi"("Raw Data From DB Actor"=w306, "error in (no error)"=w307, "ERP-Inventory in"=w308) -> ("error out"=w305:errorcluster, "ERP-Inventory out"=w304:refnum<class "ERP-Inventory.lvclass">)  [unwired: 7 in]
      }
      frame "DBActor: Refresh Pull Inventory" {
        n109 = call "JSON-ActorCommand.vi"("Payload"="", "error in"=w330, "Reply Command"="ReplyWithQuery" ("Value"), "SQL Statement"="Where Status='Ready To Be Picked'" ("Value"), "Table"="WorkOrders") -> ("error out"=w327:errorcluster, "Output JSON Object"=w325:string)  [unwired: 5 in]
        n110 = call "PCert-ConfigPageNF-AskDB.vi"("Timeout"=500, "error in (no error)"=w327, "Request Body"=w325, "Request Header"="Query" ("Message Header"), "ERP-ConfigPageNF in"=w326) -> ("error out"=w322:errorcluster, "ERP-ConfigPageNF out"=w323:refnum<class "ERP-Inventory.lvclass">, "Raw Data From DB"=w324:string[][])  [unwired: 2 in, 2 out]
        n111 = call "Inventory-PullInventoryTree.vi"("Raw Data From DB Actor"=w324, "error in (no error)"=w322, "ERP-Inventory in"=w323) -> ("error out"=w320:errorcluster, "ERP-Inventory out"=w321:refnum<class "ERP-Inventory.lvclass">)  [unwired: 7 in]
      }
      frame "Actor: Add Finished Goods" {
        w337 = 1 ("Column Number")
        n112 = property on="Part Numbers" class="Ring (strict)"(error in=w342) -> (error out=w341:errorcluster, "Strings []"=w359:string[], "Value"=w358:u16)  [unwired: 1 in, 1 out]
        n113 = Index Array(array=w359, index=w358) -> (element=w339:string)
        n114 = call "Inventory-Add#toIventory.vi"("Quanity to Add/Subtract"="Quanity to Add/Subtract", "error in (no error)"=w341, "Part Number In"=w339, "ERP-Inventory in"=w360) -> ("error out"=w338:errorcluster, "Add-Converted to String"=w336:string, "ERP-Inventory out"=w355:refnum<class "ERP-Inventory.lvclass">, "Part Number Out"=w340:string)  [unwired: 4 in]
        n115 = Concatenate Strings("Where Assembled_Part_Number='" ("SQL Statement"), w340, "'" ("string")) -> (w349:string)
        n116 = call "LVtoJSON-DBUpdate.vi"("Datatype"=0, "Column Number"=w337, "Payload"=w336, "Update All"=FALSE, "error in"=w338, "SQL Statement"=w349, "Table"="Inventory") -> ("error out"=w351:errorcluster, "Output JSON Object"=w350:string)  [unwired: 3 in]
        n117 = Equal?(x=w339, y="") -> (x = y?=w344:bool)
        n118 = case shown="False" w344 {
          tunnel: w355 -> [w371 w385]
          tunnel: [w375 w385] -> w354
          tunnel: [w362 w384] -> w353
          tunnel: w351 -> [w370 w384]
          tunnel: w350 -> [w369 _]
          tunnel: "Please Choose a part number to update from the drop down menu. \n\nTry again!" ("message") -> [_ w383]
          tunnel: w337 -> [w367 _]
          tunnel: w336 -> [w366 _]
          frame False {
            n119 = call "PCert-ConfigPageNF-AskDB.vi"("Timeout"=500, "error in (no error)"=w370, "Request Body"=w369, "Request Header"="Update" ("Message Header"), "ERP-ConfigPageNF in"=w371) -> ("error out"=w365:errorcluster, "ERP-ConfigPageNF out"=w372:refnum<class "ERP-Inventory.lvclass">, "Raw Data From DB"=w368:string[][])  [unwired: 2 in, 2 out]
            n120 = call "Inventory-UpdateSuccess.vi"("Raw Data From DB Actor"=w368, "Column#"=w367, "Data"=w366, "error in"=w365) -> ("Update Transaction Complete"=w364:bool, "error out"=w363:errorcluster)  [unwired: 10 in]
            n121 = case shown="True" w364 {
              tunnel: [w376 w381] -> w375
              tunnel: w372 -> [w376 w380]
              tunnel: w363 -> [w377 w379]
              tunnel: [w377 w379] -> w362
              frame False {
                n122 = One Button Dialog(message="The Database did not update. Please try the transaction again") -> ()  [unwired: 1 in, 1 out]
              }
              frame True {
                n123 = call "FTW-Actor-AddJob-Next.vi"("Add Next in Job Queue"="DBActor: Refresh Finished Goods", "FTW Actor Instance"=w380) -> ("FTW Actor Instance out"=w381:refnum<class "ERP-Inventory.lvclass">)  [unwired: 2 in]
              }
            }
          }
          frame True {
            n124 = One Button Dialog(message=w383) -> ()  [unwired: 1 in, 1 out]
          }
        }
      }
      frame "Actor: Add Raw Goods" {
        w391 = 1 ("Column Number")
        n125 = property on="Part Numbers_Raw Goods" class="Ring (strict)"(error in=w388) -> (error out=w408:errorcluster, "Strings []"=w409:string[], "Value"=w410:u16)  [unwired: 1 in, 1 out]
        n126 = Index Array(array=w409, index=w410) -> (element=w393:string)
        n127 = call "Inventory-Add#toIventory.vi"("Quanity to Add/Subtract"="Quanity to Add/Subtract_Raw Goods", "error in (no error)"=w408, "Part Number In"=w393, "ERP-Inventory in"=w389) -> ("error out"=w392:errorcluster, "Add-Converted to String"=w390:string, "ERP-Inventory out"=w404:refnum<class "ERP-Inventory.lvclass">, "Part Number Out"=w394:string)  [unwired: 4 in]
        n128 = Concatenate Strings("Where Raw_Good_PartNumber='" ("SQL Statement"), w394, "'" ("string")) -> (w401:string)
        n129 = call "LVtoJSON-DBUpdate.vi"("Datatype"=0, "Column Number"=w391, "Payload"=w390, "Update All"=FALSE, "error in"=w392, "SQL Statement"=w401, "Table"="RawGoodInventory") -> ("error out"=w403:errorcluster, "Output JSON Object"=w402:string)  [unwired: 3 in]
        n130 = Equal?(x=w393, y="") -> (x = y?=w396:bool)
        n131 = case shown="False" w396 {
          tunnel: w404 -> [w421 w435]
          tunnel: [w425 w435] -> w387
          tunnel: [w412 w434] -> w386
          tunnel: w403 -> [w420 w434]
          tunnel: w402 -> [w419 _]
          tunnel: "Please Choose a part number to update from the drop down menu. \n\nTry again!" ("message") -> [_ w433]
          tunnel: w391 -> [w417 _]
          tunnel: w390 -> [w416 _]
          frame False {
            n132 = call "PCert-ConfigPageNF-AskDB.vi"("Timeout"=500, "error in (no error)"=w420, "Request Body"=w419, "Request Header"="Update" ("Message Header"), "ERP-ConfigPageNF in"=w421) -> ("error out"=w415:errorcluster, "ERP-ConfigPageNF out"=w422:refnum<class "ERP-Inventory.lvclass">, "Raw Data From DB"=w418:string[][])  [unwired: 2 in, 2 out]
            n133 = call "Inventory-UpdateSuccess.vi"("Raw Data From DB Actor"=w418, "Column#"=w417, "Data"=w416, "error in"=w415) -> ("Update Transaction Complete"=w414:bool, "error out"=w413:errorcluster)  [unwired: 10 in]
            n134 = case shown="True" w414 {
              tunnel: [w426 w431] -> w425
              tunnel: w422 -> [w426 w430]
              tunnel: w413 -> [w427 w429]
              tunnel: [w427 w429] -> w412
              frame False {
                n135 = One Button Dialog(message="The Database did not update. Please try the transaction again") -> ()  [unwired: 1 in, 1 out]
              }
              frame True {
                n136 = call "FTW-Actor-AddJob-Next.vi"("Add Next in Job Queue"="DBActor: Refresh Raw Goods", "FTW Actor Instance"=w430) -> ("FTW Actor Instance out"=w431:refnum<class "ERP-Inventory.lvclass">)  [unwired: 2 in]
              }
            }
          }
          frame True {
            n137 = One Button Dialog(message=w433) -> ()  [unwired: 1 in, 1 out]
          }
        }
      }
      frame "Actor: Subtract Finished Goods" {
        w440 = 1 ("Column Number")
        n138 = local read "Quanity to Add/Subtract"() -> (w458:i32)
        n139 = property on="Part Numbers" class="Ring (strict)"(error in=w439) -> (error out=w460:errorcluster, "Strings []"=w453:string[], "Value"=w452:u16)  [unwired: 1 in, 1 out]
        n140 = Index Array(array=w453, index=w452) -> (element=w459:string)
        n141 = call "Inventory-Subtract#FromIventory.vi"("Quanity to Add/Subtract"=w458, "error in (no error)"=w460, "Part Number In"=w459, "ERP-Inventory in"=w438) -> ("error out"=w455:errorcluster, "Subtract-Converted to String"=w456:string, "ERP-Inventory out"=w454:refnum<class "ERP-Inventory.lvclass">, "Part Number Out"=w457:string)  [unwired: 4 in]
        n142 = Concatenate Strings("Where Assembled_Part_Number='" ("SQL Statement"), w457, "'" ("string")) -> (w447:string)
        n143 = call "LVtoJSON-DBUpdate.vi"("Datatype"=0, "Column Number"=w440, "Payload"=w456, "Update All"=FALSE, "error in"=w455, "SQL Statement"=w447, "Table"="Inventory") -> ("error out"=w449:errorcluster, "Output JSON Object"=w448:string)  [unwired: 3 in]
        n144 = Equal?(x=w459, y="") -> (x = y?=w442:bool)
        n145 = case shown="False" w442 {
          tunnel: w454 -> [w471 w485]
          tunnel: [w475 w485] -> w436
          tunnel: [w462 w484] -> w437
          tunnel: w449 -> [w470 w484]
          tunnel: w448 -> [w469 _]
          tunnel: "Please Choose a part number to update from the drop down menu. \n\nTry again!" ("message") -> [_ w483]
          tunnel: w440 -> [w467 _]
          tunnel: w456 -> [w466 _]
          frame False {
            n146 = call "PCert-ConfigPageNF-AskDB.vi"("Timeout"=500, "error in (no error)"=w470, "Request Body"=w469, "Request Header"="Update" ("Message Header"), "ERP-ConfigPageNF in"=w471) -> ("error out"=w465:errorcluster, "ERP-ConfigPageNF out"=w472:refnum<class "ERP-Inventory.lvclass">, "Raw Data From DB"=w468:string[][])  [unwired: 2 in, 2 out]
            n147 = call "Inventory-UpdateSuccess.vi"("Raw Data From DB Actor"=w468, "Column#"=w467, "Data"=w466, "error in"=w465) -> ("Update Transaction Complete"=w464:bool, "error out"=w463:errorcluster)  [unwired: 10 in]
            n148 = case shown="True" w464 {
              tunnel: [w476 w481] -> w475
              tunnel: w472 -> [w476 w480]
              tunnel: w463 -> [w477 w479]
              tunnel: [w477 w479] -> w462
              frame False {
                n149 = One Button Dialog(message="The Database did not update. Please try the transaction again") -> ()  [unwired: 1 in, 1 out]
              }
              frame True {
                n150 = call "FTW-Actor-AddJob-Next.vi"("Add Next in Job Queue"="DBActor: Refresh Finished Goods", "FTW Actor Instance"=w480) -> ("FTW Actor Instance out"=w481:refnum<class "ERP-Inventory.lvclass">)  [unwired: 2 in]
              }
            }
          }
          frame True {
            n151 = One Button Dialog(message=w483) -> ()  [unwired: 1 in, 1 out]
          }
        }
      }
      frame "Actor: Subtract Raw Goods" {
        w490 = 1 ("Column Number")
        n152 = local read "Quanity to Add/Subtract_Raw Goods"() -> (w506:i32)
        n153 = property on="Part Numbers_Raw Goods" class="Ring (strict)"(error in=w489) -> (error out=w504:errorcluster, "Strings []"=w502:string[], "Value"=w503:u16)  [unwired: 1 in, 1 out]
        n154 = Index Array(array=w502, index=w503) -> (element=w505:string)
        n155 = call "Inventory-Subtract#FromIventory.vi"("Quanity to Add/Subtract"=w506, "error in (no error)"=w504, "Part Number In"=w505, "ERP-Inventory in"=w488) -> ("error out"=w509:errorcluster, "Subtract-Converted to String"=w510:string, "ERP-Inventory out"=w508:refnum<class "ERP-Inventory.lvclass">, "Part Number Out"=w507:string)  [unwired: 4 in]
        n156 = Concatenate Strings("Where Raw_Good_PartNumber='" ("SQL Statement"), w507, "'" ("string")) -> (w497:string)
        n157 = call "LVtoJSON-DBUpdate.vi"("Datatype"=0, "Column Number"=w490, "Payload"=w510, "Update All"=FALSE, "error in"=w509, "SQL Statement"=w497, "Table"="RawGoodInventory") -> ("error out"=w499:errorcluster, "Output JSON Object"=w498:string)  [unwired: 3 in]
        n158 = Equal?(x=w505, y="") -> (x = y?=w492:bool)
        n159 = case shown="False" w492 {
          tunnel: w508 -> [w521 w535]
          tunnel: [w525 w535] -> w487
          tunnel: [w512 w534] -> w486
          tunnel: w499 -> [w520 w534]
          tunnel: w498 -> [w519 _]
          tunnel: "Please Choose a part number to update from the drop down menu. \n\nTry again!" ("message") -> [_ w533]
          tunnel: w490 -> [w517 _]
          tunnel: w510 -> [w516 _]
          frame False {
            n160 = call "PCert-ConfigPageNF-AskDB.vi"("Timeout"=500, "error in (no error)"=w520, "Request Body"=w519, "Request Header"="Update" ("Message Header"), "ERP-ConfigPageNF in"=w521) -> ("error out"=w515:errorcluster, "ERP-ConfigPageNF out"=w522:refnum<class "ERP-Inventory.lvclass">, "Raw Data From DB"=w518:string[][])  [unwired: 2 in, 2 out]
            n161 = call "Inventory-UpdateSuccess.vi"("Raw Data From DB Actor"=w518, "Column#"=w517, "Data"=w516, "error in"=w515) -> ("Update Transaction Complete"=w514:bool, "error out"=w513:errorcluster)  [unwired: 10 in]
            n162 = case shown="True" w514 {
              tunnel: [w526 w531] -> w525
              tunnel: w522 -> [w526 w530]
              tunnel: w513 -> [w527 w529]
              tunnel: [w527 w529] -> w512
              frame False {
                n163 = One Button Dialog(message="The Database did not update. Please try the transaction again") -> ()  [unwired: 1 in, 1 out]
              }
              frame True {
                n164 = call "FTW-Actor-AddJob-Next.vi"("Add Next in Job Queue"="DBActor: Refresh Raw Goods", "FTW Actor Instance"=w530) -> ("FTW Actor Instance out"=w531:refnum<class "ERP-Inventory.lvclass">)  [unwired: 2 in]
              }
            }
          }
          frame True {
            n165 = One Button Dialog(message=w533) -> ()  [unwired: 1 in, 1 out]
          }
        }
      }
      frame "Actor: Add New Finished Goods Part#" {
        n166 = Unbundle By Name(w559) -> ("New Inventory Assembled Part Number to Add"=w538:string, "Quanity to Add To Inventory New Part"=w547:i32, "Minimum Number Allowed \nIn Inventory"=w545:i32, "Maximum Number Allowed\nIn Inventory"=w544:i32)
        n167 = property on="Part Numbers" class="Ring (strict)"(error in=w558) -> (error out=w554:errorcluster, "Strings []"=w557:string[])  [unwired: 1 in, 1 out]
        n168 = Array Size(array=w557) -> (size(s)=w556:i32)
        n169 = To Upper Case(1:w538) -> (0:w537:string)
        n170 = Number To Decimal String(number=w547) -> (decimal integer string=w546:string)  [unwired: 1 in]
        n171 = Number To Decimal String(number=w545) -> (decimal integer string=w543:string)  [unwired: 1 in]
        n172 = Number To Decimal String(number=w544) -> (decimal integer string=w542:string)  [unwired: 1 in]
        n173 = Insert Into Array(array=w557, index=w556, new element=w537) -> (w555:string[])
        n174 = property on="Part Numbers" class="Ring (strict)"(error in=w554, "Strings []"=w555) -> (error out=w550:errorcluster)  [unwired: 1 in, 1 out]
        n175 = Bundle(cluster=T8 {"New Inventory Assembled Part Number to Add"="", "On the Shelf"="", "Minimum"="", "Maximum"=""}, "New Inventory Assembled Part Number to Add"=w537, "On the Shelf"=w546, "Minimum"=w543, "Maximum"=w542) -> (w540:T8)
        n176 = Flatten To JSON(anything=w540, error in (no error)=w550) -> (JSON string=w548:string, 11:w549:errorcluster)  [unwired: 1 in]
        n177 = call "LVtoJSON-DBInsert.vi"("Type Of Insertion"=0, "Payload"=w548, "error in"=w549, "Table"="Inventory") -> ("error out"=w552:errorcluster, "Output JSON Object"=w551:string)  [unwired: 6 in]
        n178 = call "PCert-ConfigPageNF-TellDB.vi"("Timeout"=500, "error in (no error)"=w552, "Message Body"=w551, "Message Header"="Insert", "ERP-ConfigPageNF in"=w559) -> ("error out"=w536:errorcluster, "ERP-ConfigPageNF out"=w561:refnum<class "ERP-Inventory.lvclass">)  [unwired: 5 in]
        n179 = call "FTW-Actor-AddJob-Next.vi"("Add Next in Job Queue"="DBActor: Refresh Finished Goods", "FTW Actor Instance"=w561) -> ("FTW Actor Instance out"=w564:refnum<class "ERP-Inventory.lvclass">)  [unwired: 2 in]
      }
      frame "Actor: Add New Raw Goods Part#" {
        n180 = Unbundle By Name(w569) -> ("New Inventory Assembled Part Number to Add"=w571:string, "Quanity to Add To Inventory New Part"=w580:i32, "Minimum Number Allowed \nIn Inventory"=w578:i32, "Maximum Number Allowed\nIn Inventory"=w577:i32)
        n181 = property on="Part Numbers_Raw Goods" class="Ring (strict)"(error in=w567) -> (error out=w587:errorcluster, "Strings []"=w590:string[])  [unwired: 1 in, 1 out]
        n182 = Array Size(array=w590) -> (size(s)=w589:i32)
        n183 = To Upper Case(1:w571) -> (0:w570:string)
        n184 = Number To Decimal String(number=w580) -> (decimal integer string=w579:string)  [unwired: 1 in]
        n185 = Number To Decimal String(number=w578) -> (decimal integer string=w576:string)  [unwired: 1 in]
        n186 = Number To Decimal String(number=w577) -> (decimal integer string=w575:string)  [unwired: 1 in]
        n187 = Insert Into Array(array=w590, index=w589, new element=w570) -> (w588:string[])
        n188 = property on="Part Numbers_Raw Goods" class="Ring (strict)"(error in=w587, "Strings []"=w588) -> (error out=w583:errorcluster)  [unwired: 1 in, 1 out]
        n189 = Bundle(cluster=T8 {"New Inventory Assembled Part Number to Add"="", "On the Shelf"="", "Minimum"="", "Maximum"=""}, "New Inventory Assembled Part Number to Add"=w570, "On the Shelf"=w579, "Minimum"=w576, "Maximum"=w575) -> (w573:T8)
        n190 = Flatten To JSON(anything=w573, error in (no error)=w583) -> (JSON string=w581:string, 11:w582:errorcluster)  [unwired: 1 in]
        n191 = call "LVtoJSON-DBInsert.vi"("Type Of Insertion"=0, "Payload"=w581, "error in"=w582, "Table"="Inventory") -> ("error out"=w585:errorcluster, "Output JSON Object"=w584:string)  [unwired: 6 in]
        n192 = call "PCert-ConfigPageNF-TellDB.vi"("Timeout"=500, "error in (no error)"=w585, "Message Body"=w584, "Message Header"="Insert", "ERP-ConfigPageNF in"=w569) -> ("error out"=w566:errorcluster, "ERP-ConfigPageNF out"=w592:refnum<class "ERP-Inventory.lvclass">)  [unwired: 5 in]
        n193 = call "FTW-Actor-AddJob-Next.vi"("Add Next in Job Queue"="DBActor: Refresh Raw Goods", "FTW Actor Instance"=w592) -> ("FTW Actor Instance out"=w568:refnum<class "ERP-Inventory.lvclass">)  [unwired: 2 in]
      }
      frame "Actor: Delete Finished Goods Part#" {
        n194 = property on="Finish Good Part# to Delete" class="Ring (strict)"(error in=w604) -> (error out=w603:errorcluster, "Strings []"=w607:string[], "Value"=w606:u16)  [unwired: 1 in, 1 out]
        n195 = Index Array(array=w607, index=w606) -> (element=w599:string)
        n196 = Delete From Array(array=w607, index=w606) -> (array with subset deleted=w605:string[])  [unwired: 1 in, 1 out]
        n197 = property on="Finish Good Part# to Delete" class="Ring (strict)"(error in=w603, "Strings []"=w605) -> (error out=w602:errorcluster)  [unwired: 1 in, 1 out]
        n198 = property on="Part Numbers" class="Ring (strict)"(error in=w602, "Strings []"=w605) -> (error out=w601:errorcluster)  [unwired: 1 in, 1 out]
        n199 = To Upper Case(1:w599) -> (0:w598:string)
        n200 = Concatenate Strings("Where Assembled_Part_Number ='" ("SQL Statement"), w598, "'" ("string")) -> (w596:string)
        n201 = call "LVtoJSON-DBInsert.vi"("Type Of Insertion"=0, "error in"=w601, "SQL Statement"=w596, "Table"="Inventory") -> ("error out"=w613:errorcluster, "Output JSON Object"=w612:string)  [unwired: 6 in]
        n202 = call "PCert-ConfigPageNF-TellDB.vi"("Timeout"=500, "error in (no error)"=w613, "Message Body"=w612, "Message Header"="Delete", "ERP-ConfigPageNF in"=w610) -> ("error out"=w608:errorcluster, "ERP-ConfigPageNF out"=w616:refnum<class "ERP-Inventory.lvclass">)  [unwired: 5 in]
        n203 = call "FTW-Actor-AddJob-Next.vi"("Add Next in Job Queue"="DBActor: Refresh Finished Goods", "FTW Actor Instance"=w616) -> ("FTW Actor Instance out"=w609:refnum<class "ERP-Inventory.lvclass">)  [unwired: 2 in]
      }
      frame "Actor: Delete Raw Goods Part#" {
        n204 = property on="Raw Goods Part # to Delete" class="Ring (strict)"(error in=w624) -> (error out=w623:errorcluster, "Strings []"=w626:string[], "Value"=w625:u16)  [unwired: 1 in, 1 out]
        n205 = Index Array(array=w626, index=w625) -> (element=w630:string)
        n206 = Delete From Array(array=w626, index=w625) -> (array with subset deleted=w622:string[])  [unwired: 1 in, 1 out]
        n207 = property on="Raw Goods Part # to Delete" class="Ring (strict)"(error in=w623, "Strings []"=w622) -> (error out=w621:errorcluster)  [unwired: 1 in, 1 out]
        n208 = property on="Part Numbers_Raw Goods" class="Ring (strict)"(error in=w621, "Strings []"=w622) -> (error out=w620:errorcluster)  [unwired: 1 in, 1 out]
        n209 = To Upper Case(1:w630) -> (0:w629:string)
        n210 = Concatenate Strings("Where Raw_Good_PartNumber ='" ("SQL Statement"), w629, "'" ("string")) -> (w627:string)
        n211 = call "LVtoJSON-DBInsert.vi"("Type Of Insertion"=0, "error in"=w620, "SQL Statement"=w627, "Table"="Inventory") -> ("error out"=w637:errorcluster, "Output JSON Object"=w636:string)  [unwired: 6 in]
        n212 = call "PCert-ConfigPageNF-TellDB.vi"("Timeout"=500, "error in (no error)"=w637, "Message Body"=w636, "Message Header"="Delete", "ERP-ConfigPageNF in"=w634) -> ("error out"=w632:errorcluster, "ERP-ConfigPageNF out"=w640:refnum<class "ERP-Inventory.lvclass">)  [unwired: 5 in]
        n213 = call "FTW-Actor-AddJob-Next.vi"("Add Next in Job Queue"="DBActor: Refresh Finished Goods", "FTW Actor Instance"=w640) -> ("FTW Actor Instance out"=w633:refnum<class "ERP-Inventory.lvclass">)  [unwired: 2 in]
      }
      frame "==========Tree Jobs==========" {
      }
      frame "Tree: FulFill Iventory WO" {
      }
      frame "==========WO Note Creation==========" {
      }
      frame "Note: Create New Stock Inventory Note" {
      }
      frame "Note: View/Edit Stock Inventory Note" {
      }
      frame "Note: Create New Pull WO Inventory Note" {
      }
      frame "Note: Edit/View Pull WO Inventory Note" {
      }
    }
    n214 = call "FTW-Actor-CheckShutdown.vi"("FTW Actor Instance"=w16, "error in"=w14) -> ("FTW Actor Instance out"=w15:refnum<class "ERP-Inventory.lvclass">, "Shutdown?"=w12:bool, "error out"=w13:errorcluster)  [unwired: 11 in]
  }
  n215 = call-dynamic "FTW-Actor-Destroy.vi"("FTW Actor Instance"=w9, "error in"=w8) -> ("error out"=w2:errorcluster)  [unwired: 13 in]
  n216 = call "FTW-ERR-Clear.vi"("error to snuff"=w2) -> ("no error"=→"Error":errorcluster)
